vi "EnableWFGOutput.vi"(0 "object in":refnum<class "AD2andExtAWG.lvclass">, 2 "OutputEnable 2":T1, 5 "error in (no error)":errorcluster) -> (14 "object out":refnum<class "AD2andExtAWG.lvclass">, 19 "error out":errorcluster)   [LabVIEW 2019, in "AD2andExtAWG.lvclass"]
uses:
  AD2andExtAWG.lvclass
  AD2andExtAWG.lvclass/AD2andExtAWG.ctl
  AFG3022B_class/AFG3022B.lvclass
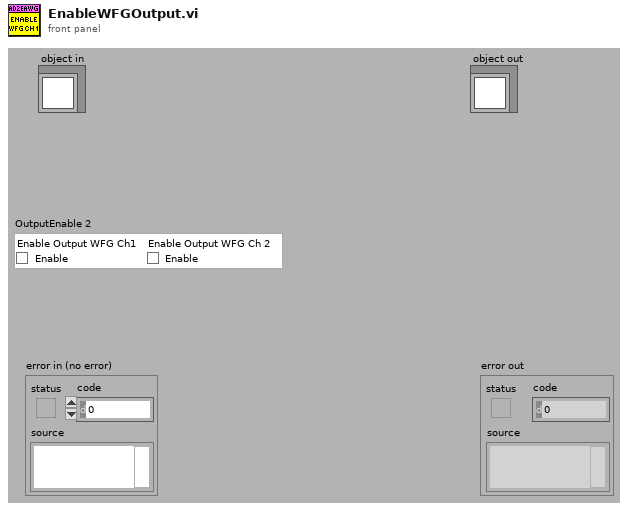
[diagram p1: front panel]
types:
  T1 = cluster{"Enable Output WFG Ch1":bool, "Enable Output WFG Ch 2":bool}
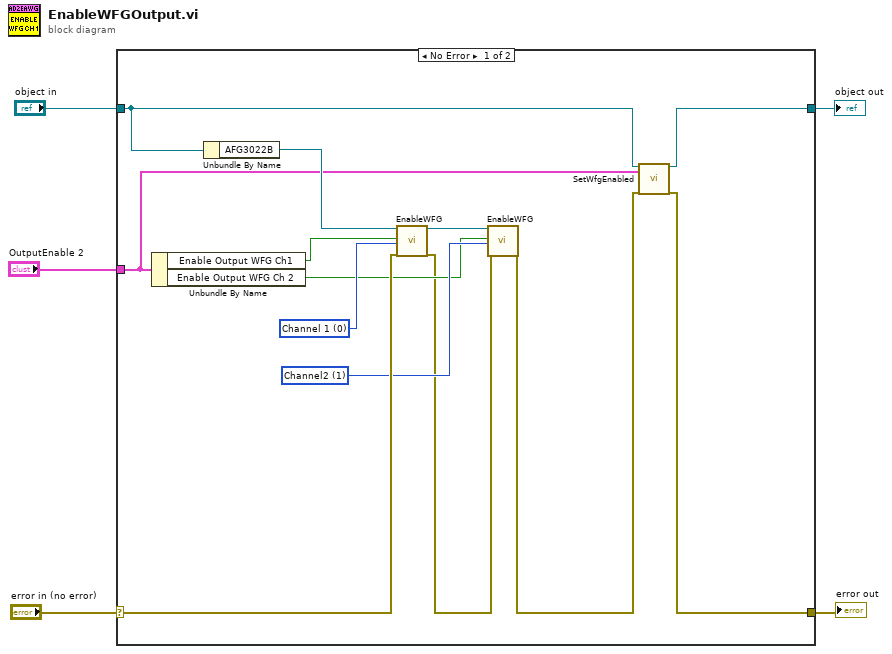
[diagram p0: block diagram]
diagram:
  n1 = case shown="No Error" "error in (no error)" {
    selector: "error in (no error)" -> [w17 w20]
    tunnel: [w6 w20] -> w4
    tunnel: [w10 w19] -> w2
    tunnel: "object in" -> [w9 w19]
    tunnel: "OutputEnable 2" -> [w8 _]
    frame No Error {
      w14 = u16 1 items=["Channel 1", "Channel2"] ("Channel (0: Channel 1)")
      w16 = u16 0 items=["Channel 1", "Channel2"] ("Channel (0: Channel 1)")
      n2 = Unbundle By Name(w8) -> ("Enable Output WFG Ch1"=w13:bool, "Enable Output WFG Ch 2"=w12:bool)
      n3 = Unbundle By Name(w9) -> ("AFG3022B"=w18:refnum<class "AFG3022B.lvclass">)
      n4 = call-dynamic "EnableWFG.vi"("object in"=w18, "Enable Output (T: Enable)"=w13, "Channel (0: Channel 1)"=w16, "error in (no error)"=w17) -> ("object out"=w15:refnum<class "AFG3022B.lvclass">, "error out"=w11:errorcluster)  [unwired: 14 in]
      n5 = call-dynamic "EnableWFG.vi"("object in"=w15, "Enable Output (T: Enable)"=w12, "Channel (0: Channel 1)"=w14, "error in (no error)"=w11) -> ("error out"=w7:errorcluster)  [unwired: 14 in, 1 out]
      n6 = call-dynamic "SetWfgEnabled.vi"("object in"=w9, "WfgEnabled"=w8, "error in (no error)"=w7) -> ("object out"=w10:refnum<class "AD2andExtAWG.lvclass">, "error out"=w6:errorcluster)  [unwired: 15 in]
    }
    frame Error {
    }
  }
  "error out" <- w4
  "object out" <- w2
